vi "MoveWindow.vi"(4 "Window Reference":refnum<vi>, 6 "Iteration":i32, 8 "error in (no error)":errorcluster, 10 "axis info in":T2, 11 "Refnum in":refnum<k1>) -> (0 "error out":errorcluster, 1 "button info":T1, 2 "axis info":T2, 3 "Refnum out":refnum<k1>)   [LabVIEW 2014, in "SmartPalette.lvlib"]
uses:
  <vilib>/Utility/inputDevices.llb/mouseAcquire.vi
  SmartPalette.lvlib
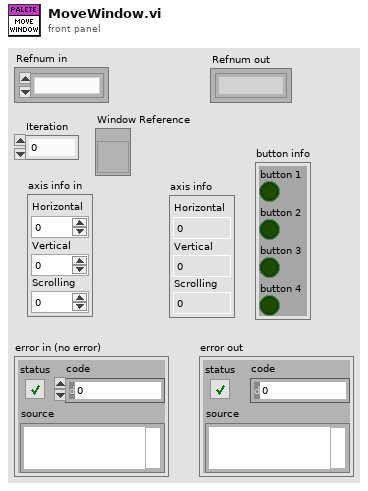
[diagram p1: front panel]
types:
  T1 = cluster{"button 1":bool, "button 2":bool, "button 3":bool, "button 4":bool}
  T2 = cluster{"Horizontal":i32, "Vertical":i32, "Scrolling":i32}
  T3 = typedef "LVRectTypeDef.ctl" = cluster{"Left":i16, "Top":i16, "Right":i16, "Bottom":i16}
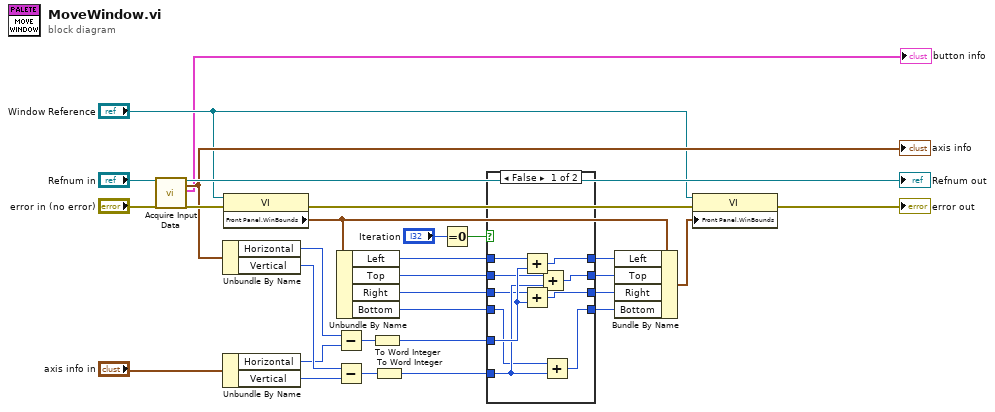
[diagram p0: block diagram]
diagram:
  n1 = call-poly <vilib>:"Acquire Input Data.vi"("device ID"="Refnum in", "error in (no error)"="error in (no error)") -> ("device ID"=→"Refnum out":refnum<k1>, "axis info"=w26:T2, "button info"=→"button info":T1, "error out"=w27:errorcluster)  [unwired: 1 in, 13 out]
  "axis info" <- w26
  n2 = Unbundle By Name(w26) -> ("Horizontal"=w9:i32, "Vertical"=w11:i32)
  n3 = Unbundle By Name("axis info in") -> ("Horizontal"=w10:i32, "Vertical"=w12:i32)
  n4 = property class="VI"(reference="Window Reference", error in=w27) -> (error out=w6:errorcluster, "Front Panel.WinBounds"=w4:T3)  [unwired: 1 out]
  n5 = Subtract(x=w9, y=w10) -> (x-y=w13:i32)
  n6 = Subtract(x=w11, y=w12) -> (x-y=w14:i32)
  n7 = Unbundle By Name(w4) -> ("Left"=w16:i16, "Top"=w17:i16, "Right"=w18:i16, "Bottom"=w19:i16)
  n8 = To Word Integer(number=w13) -> (16bit integer=w29:i16)
  n9 = To Word Integer(number=w14) -> (16bit integer=w30:i16)
  n10 = Equal To 0?(x="Iteration") -> (x = 0?=w8:bool)
  n11 = case shown="False" w8 {
    tunnel: w29 -> [w40 _]
    tunnel: w30 -> [w39 _]
    tunnel: w16 -> [w33 w41]
    tunnel: w17 -> [w36 w42]
    tunnel: w18 -> [w34 w43]
    tunnel: w19 -> [w35 w44]
    tunnel: [w38 w44] -> w20
    tunnel: [w31 w43] -> w21
    tunnel: [w37 w42] -> w22
    tunnel: [w32 w41] -> w23
    frame False {
      n12 = Add(x=w33, y=w40) -> (x+y=w32:i16)
      n13 = Add(x=w34, y=w40) -> (x+y=w31:i16)
      n14 = Add(x=w36, y=w39) -> (x+y=w37:i16)
      n15 = Add(x=w35, y=w39) -> (x+y=w38:i16)
    }
    frame True {
    }
  }
  n16 = Bundle By Name(cluster=w4, "Left"=w23, "Top"=w22, "Right"=w21, "Bottom"=w20) -> (w5:T3)
  n17 = property class="VI"(reference="Window Reference", error in=w6, "Front Panel.WinBounds"=w5) -> (error out=→"error out":errorcluster)  [unwired: 1 out]
